vi "Thermistor_Temp_Stamp.vi"(8 "error in":errorcluster, 11 "DataCluster":T1={"Core"={"Current VI Reference"=refnum, "Close Panel on Exit?"=FALSE, "Exit"=FALSE}, "Connections"={"cDAQ Therm"={"Task"="ThermTask", "Connected"=FALSE, "Active"=FALSE}, "cDAQ Voltage"={"Task"="", "Connected"=FALSE, "Active"=FALSE}, "Camera"={"Session"="", "Connected"=FALSE, "Active"=FALSE}}, "Data Acquisition"={"Setup"={"Label"="_2", "Operator"="", "Notes"="", "TempGrad"=1.0, "TargetTemp"=1.0, "Sample Volume"=1.0}, "Camera"={"Image"=refnum, "Save Image"=refnum}, "Thermistor"={"Sample Size"=1, "Calibration"={"B0.100"=[3450.0, 3450.0, 3450.0, 3450.0, 3450.0, 3450.0, 3450.0, 3450.0], "R25"=[10.74, 10.74, 10.74, 10.74, 10.74, 10.74, 10.74, 10.74], "V_S"=10.0, "R_S"=10.0}, "Timing Mode"=14713}, "Queue"={"Size"=1, "Queue"=refnum}, "Sample Rate"=1, "Active"=TRUE, "Ready"=TRUE, "Partition"={"Data"=[["A", "35%", "", "", ""], ["B", "15%", "", "", ""], ["C", "5%", "", "", ""], ["D", "35%", "", "", ""], ["E", "Test sample", "", "", ""], ["F", "High Concentration", "", "", ""], ["G", "Low Concentration", "", "", ""], ["X", "Empty", "", "", ""]], "Cell Label"="F", "Cell Color"=5095150, "Height"=8, "Width"=12, "Grid"=[["A", "A", "A", "B", "B", "B", "B", "B", "B", "B", "B", "B"], ["A", "A", "A", "B", "B", "B", "B", "B", "B", "B", "B", "B"], ["A", "A", "A", "B", "B", "B", "B", "B", "B", "B", "B", "B"], ["A", "A", "A", "C", "C", "C", "D", "D", "D", "D", "D", "D"], ["A", "A", "A", "C", "C", "C", "D", "D", "D", "D", "D", "D"], ["A", "A", "A", "C", "C", "C", "E", "E", "F", "F", "G", "G"], ["A", "A", "A", "C", "C", "C", "E", "E", "F", "F", "G", "G"], ["A", "A", "A", "C", "C", "C", "E", "E", "F", "F", "G", "G"]]}}, "Control"={"Sample Rate"=1, "PID gains"={"proportional gain (Kc)"=1.0, "integral time (Ti, min)"=0.01, "derivative time (Td, min)"=0.0}}} {"Control"."PID gains"."derivative time (Td, min)" format="%.3f"; "Control"."PID gains"."integral time (Ti, min)" format="%.3f"; "Control"."PID gains"."proportional gain (Kc)" format="%.3f"; "Control"."Sample Rate" min=1 max=20 step=1 format="%.0f Samples/sec"; "Data Acquisition"."Thermistor"."Timing Mode" items=["Automatic"=16097, "High Resolution"=10195, "High Speed"=14712, "Best 50 Hz Rejection"=14713, "Best 60 Hz Rejection"=14714, "Custom"=10137]; "Data Acquisition"."Thermistor"."Calibration"."R_S" min=0.1 max=1000.0 format="%#_g kOhm"; "Data Acquisition"."Thermistor"."Calibration"."V_S" min=5.0 max=48.0 format="%#_g V"; "Data Acquisition"."Thermistor"."Calibration"."R25" min=0.1 max=1000.0 format="%#_g kOhm"; "Data Acquisition"."Thermistor"."Calibration"."B0.100" min=100.0 max=10000.0 format="%#_g K"; "Data Acquisition"."Thermistor"."Sample Size" min=1 max=200; "Data Acquisition"."Sample Rate" min=20 max=240 format="%.0f samples/min"; "Data Acquisition"."Queue"."Size" min=1 max=200; "Data Acquisition"."Setup"."Sample Volume" min=0.0 max=500.0 format="%#_g µL"; "Data Acquisition"."Setup"."TargetTemp" min=-30.0 max=30.0 step=0.5 format="%#_g °C"; "Data Acquisition"."Setup"."TempGrad" min=-100.0 max=100.0 step=0.1 format="%#_g °C/min"}) -> (0 "error out":errorcluster, 3 "mean temp":string)   [LabVIEW 2020]
uses:
  DataCluster.ctl
  <vilib>/userDefined/High Color/IMAQdx.ctl
  <vilib>/vision/Image Controls.llb/IMAQ Image.ctl
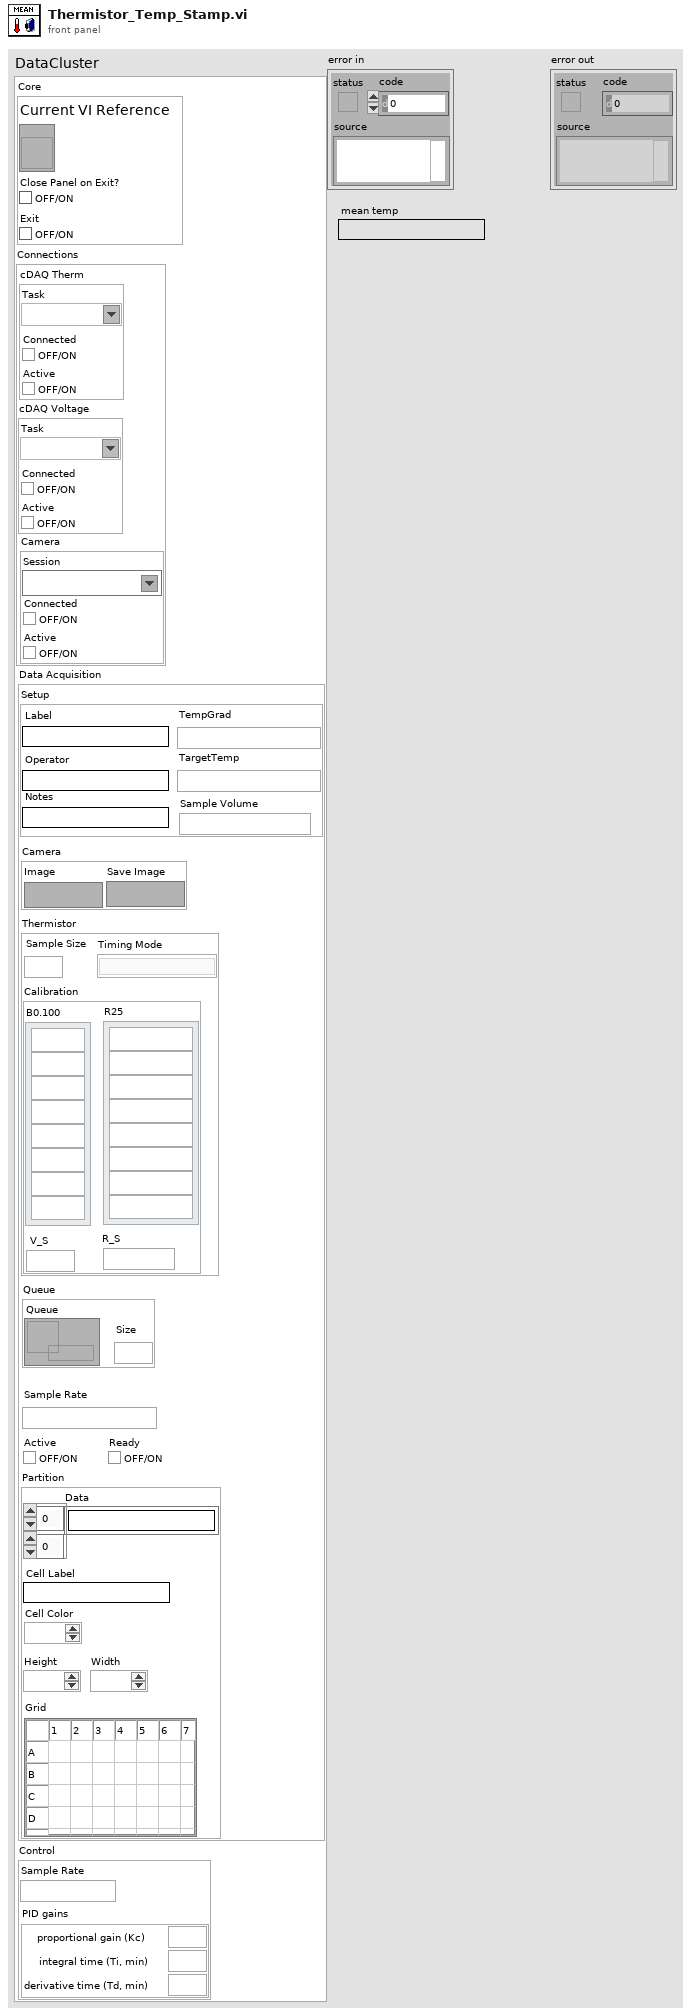
[diagram p1: front panel]
types:
  T1 = typedef "DataCluster.ctl" = cluster{"Core":cluster{"Current VI Reference":refnum<vi>, "Close Panel on Exit?":bool, "Exit":bool}, "Connections":cluster{"cDAQ Therm":cluster{"Task":refnum<k21>, "Connected":bool, "Active":bool}, "cDAQ Voltage":cluster{"Task":refnum<k21>, "Connected":bool, "Active":bool}, "Camera":cluster{"Session":T2, "Connected":bool, "Active":bool}}, "Data Acquisition":cluster{"Setup":cluster{"Label":string, "Operator":string, "Notes":string, "TempGrad":dbl, "TargetTemp":dbl, "Sample Volume":dbl}, "Camera":cluster{"Image":T3, "Save Image":T3}, "Thermistor":cluster{"Sample Size":i32, "Calibration":cluster{"B0.100":dbl[], "R25":dbl[], "V_S":dbl, "R_S":dbl}, "Timing Mode":i32}, "Queue":cluster{"Size":i32, "Queue":refnum<queue>}, "Sample Rate":i32, "Active":bool, "Ready":bool, "Partition":cluster{"Data":string[][], "Cell Label":string, "Cell Color":u32, "Height":i32, "Width":i32, "Grid":string[][]}}, "Control":cluster{"Sample Rate":i32, "PID gains":cluster{"proportional gain (Kc)":dbl, "integral time (Ti, min)":dbl, "derivative time (Td, min)":dbl}}}
  T2 = typedef "IMAQdx.ctl" = refnum<k21>
  T3 = typedef "IMAQ Image.ctl" = refnum<image>
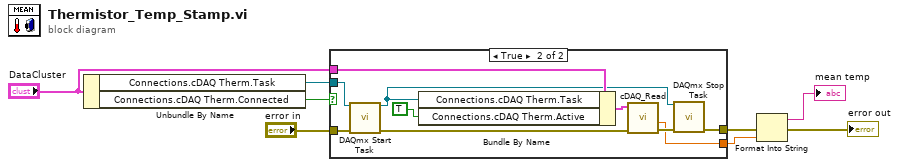
[diagram p0: block diagram]
diagram:
  n1 = Unbundle By Name("DataCluster") -> ("Connections.cDAQ Therm.Task"=w8:refnum<k21>, "Connections.cDAQ Therm.Connected"=w7:bool)
  n2 = case shown="True" w7 {
    tunnel: w8 -> [_ w19]
    tunnel: "error in" -> [w9 w18]
    tunnel: "DataCluster" -> [_ w17]
    tunnel: [w9 w11] -> w4
    tunnel: [_ w10] -> w3
    frame False {
    }
    frame True {
      n3 = call <vilib>:"DAQmx Start Task.vi"("task/channels in"=w19, "error in"=w18) -> ("task out"=w12:refnum<k21>, "error out"=w14:errorcluster)  [unwired: 12 in]
      n4 = Bundle By Name(cluster=w17, "Connections.cDAQ Therm.Task"=w12, "Connections.cDAQ Therm.Active"=TRUE) -> (w15:T1)
      n5 = call "cDAQ_Read.vi"("error in"=w14, "DataCluster"=w15) -> ("Mean Temperature"=w10:dbl, "error out"=w13:errorcluster)  [unwired: 4 in, 4 out]
      n6 = call <vilib>:"DAQmx Stop Task.vi"("task/channels in"=w12, "error in"=w13) -> ("error out"=w11:errorcluster)  [unwired: 12 in, 1 out]
    }
  }
  n7 = Format Into String(error in=w4, w3) -> (resulting string=→"mean temp":string, error out=→"error out":errorcluster)  [unwired: 2 in]
